vi "GT Add Event.vi"(8 "error in (no error)":errorcluster caption="错误输入（无错误）", 9 "pEventIndex":i16, 10 "pEvent":T1, 11 "cardNum":i16) -> (0 "error out":errorcluster caption="错误输出", 1 "pEventIndex out":i16, 2 "pEvent out":T1, 3 "function return":i16)   [LabVIEW 2020, in "gts1.lvlib"]
doc: "GT_API GT_AddEvent(short cardNum,TEvent *pEvent,short *pEventIndex);"
uses:
  gts1.lvlib
  dll/32bit/multi_card/gts.dll
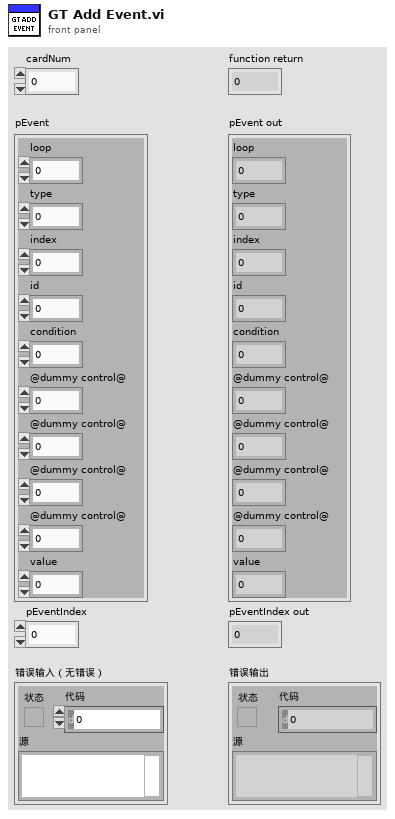
[diagram p1: front panel]
types:
  T1 = cluster{"loop":u32, "type":u16, "index":u16, "id":u16, "condition":u16, "@dummy control@":i8, "@dummy control@":i8, "@dummy control@":i8, "@dummy control@":i8, "value":dbl}
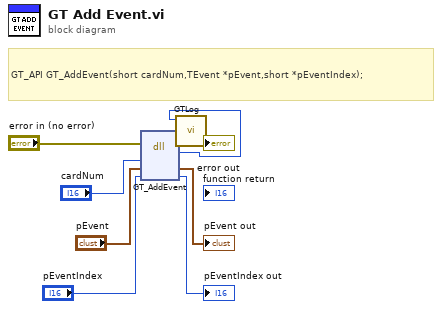
[diagram p0: block diagram]
diagram:
  # "GT_API GT_AddEvent(short cardNum,TEvent *pEvent,short *pEventIndex);"
  n1 = dll-call lib="C:/1228/dll/32bit/multi_card/gts.dll" fn="GT_AddEvent"(error in="error in (no error)", "cardNum"="cardNum", "pEvent"="pEvent", "pEventIndex"="pEventIndex") -> (error out=w3:errorcluster, w1:i16, "pEvent"=→"pEvent out":T1, "pEventIndex"=→"pEventIndex out":i16)  [unwired: 3 in, 1 out]
  n2 = call "GTLog.vi"("error in (no error)"=w3, "Numeric"=w1) -> ("error out"=→"error out":errorcluster)  [unwired: 9 in]
